vi "assembleMatrix.vi"(0 "A":dbl[][](array[numeric]), 1 "B":dbl[][](array[numeric]), 3 "C":dbl[][](array[numeric]), 4 "D":dbl[][](array[numeric])) -> (5 "ABCD":dbl[][](array[numeric]))   [LabVIEW 2014, in "NI_Gmath.lvlib"]
uses:
  NI_Gmath.lvlib
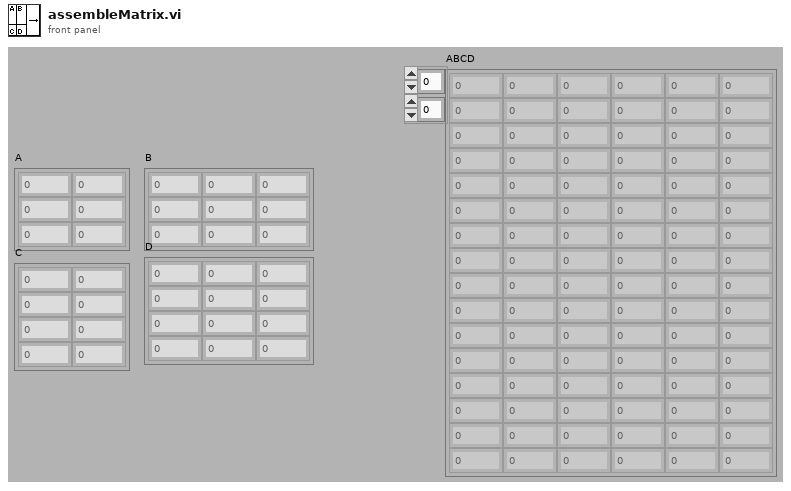
[diagram p1: front panel]
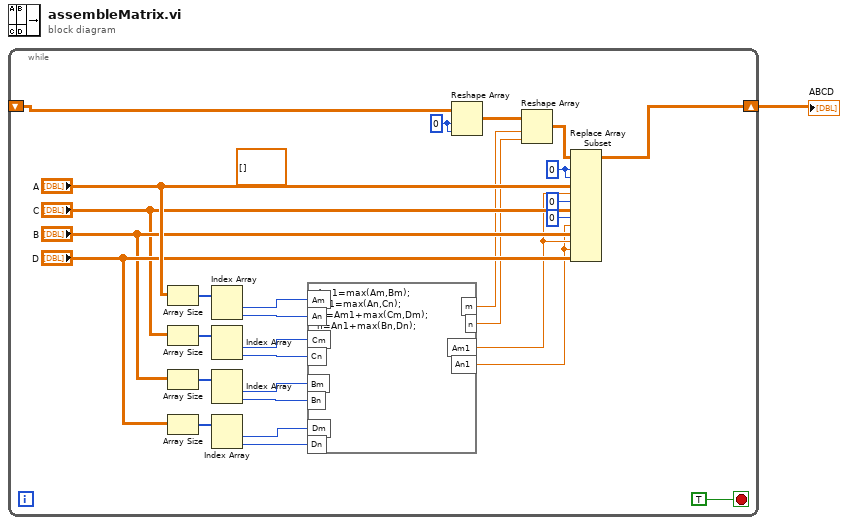
[diagram p0: block diagram]
diagram:
  n1 = while {
    shift-right: [w5] -> w1
    shift-left: _ -> [w2]
    stop <- TRUE stop-if-true
    w4 = 0 ("dimension size")
    (unwired) dbl[][] [] ("array")
    w23 = 0 ("index (row)")
    n2 = Array Size(array="A") -> (size(s)=w26:i32[])
    n3 = Array Size(array="C") -> (size(s)=w25:i32[])
    n4 = Array Size(array="B") -> (size(s)=w24:i32[])
    n5 = Array Size(array="D") -> (size(s)=w19:i32[])
    n6 = Index Array(array=w26) -> (element #1=w8:i32, element #2=w9:i32)  [unwired: 2 in]
    n7 = Index Array(array=w25) -> (element #1=w11:i32, element #2=w10:i32)  [unwired: 2 in]
    n8 = Index Array(array=w24) -> (element #1=w7:i32, element #2=w12:i32)  [unwired: 2 in]
    n9 = Index Array(array=w19) -> (element #1=w18:i32, element #2=w17:i32)  [unwired: 2 in]
    n10 = formula code="Am1=max(Am,Bm);\nAn1=max(An,Cn);\nm=Am1+max(Cm,Dm);\nn=An1+max(Bn,Dn);"("Am"=w8, "An"=w9, "Bm"=w7, "Bn"=w12, "Cm"=w11, "Cn"=w10, "Dm"=w18, "Dn"=w17) -> ("Am1"=w16:dbl, "An1"=w15:dbl, "m"=w14:dbl, "n"=w13:dbl)
    n11 = Reshape Array(w2, w4, w4) -> (w3:dbl[][])
    n12 = Reshape Array(w3, w14, w13) -> (w20:dbl[][])
    n13 = Replace Array Subset(array=w20, new element #1="A", index (row) #1=w23, index (col) #1=w23, new element #2="C", index (row) #2=w16, index (col) #2=0 ("index (row)"), new element #3="B", index (row) #3=0 ("index (row)"), index (col) #3=w15, new element #4="D", index (row) #4=w16, index (col) #4=w15) -> (w5:dbl[][])
  }
  "ABCD" <- w1
